vi "AddControlConpane__slk_mt.vi"(8 "error in (no error)":errorcluster, 11 "This VI":refnum<vi>) -> (0 "error IO":errorcluster)   [LabVIEW 2015, in "Lazyboots Menu Tool.lvlib"]
uses:
  <vilib>/SLK/Lazyboots Menu Tool/Library/Lazyboots Menu Tool.lvlib
  <vilib>/Utility/miscctls.llb/LVRectTypeDef.ctl
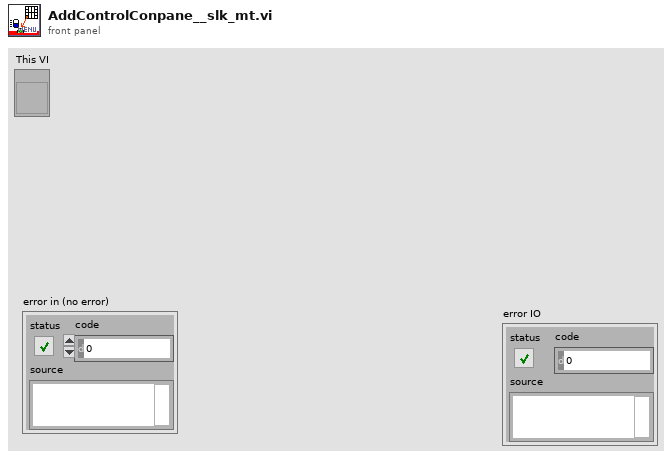
[diagram p1: front panel]
types:
  T1 = typedef "LVRectTypeDef.ctl" = cluster{"Left":i16, "Top":i16, "Right":i16, "Bottom":i16}
  T2 = typedef "LVPositionTypeDef.ctl" = cluster{"Left":i32, "Top":i32}
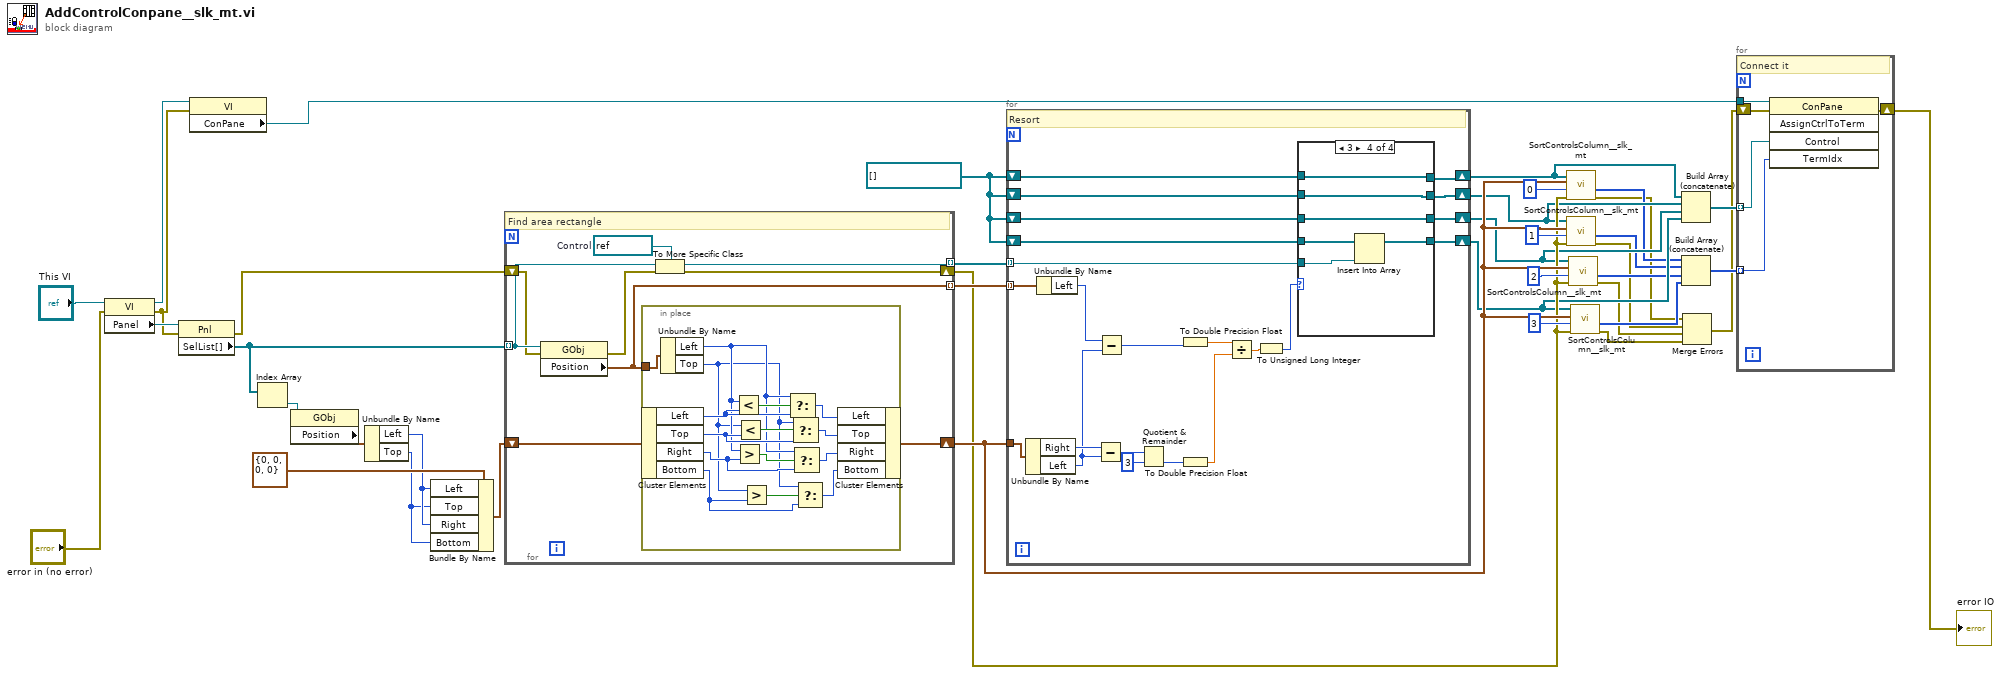
[diagram p0: block diagram]
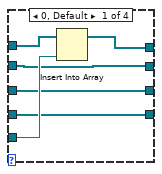
[diagram p2: hidden frame]
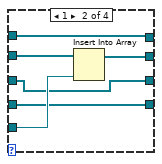
[diagram p3: hidden frame]
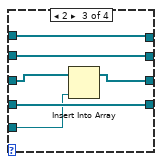
[diagram p4: hidden frame]
diagram:
  w30 = refnum<vi>[] []
  n1 = property class="VI"(reference="This VI", error in="error in (no error)") -> (reference out=w20:refnum<vi>, error out=w19:errorcluster, "Panel"=w21:refnum<vi>)
  n2 = property class="Pnl"(reference=w21, error in=w19) -> (error out=w24:errorcluster, "SelList[]"=w37:refnum<vi>[])  [unwired: 1 out]
  n3 = property class="VI"(reference=w20, error in=w19) -> ("ConPane"=w8:refnum<vi>)  [unwired: 2 out]
  n4 = Index Array(array=w37) -> (element=w36:refnum<vi>)  [unwired: 1 in]
  n5 = property class="GObj"(reference=w36) -> ("Position"=w33:T2)  [unwired: 1 in, 2 out]
  n6 = Unbundle By Name(w33) -> ("Left"=w32:i32, "Top"=w31:i32)
  n7 = Bundle By Name(cluster=T1 {"Left"=0, "Top"=0, "Right"=0, "Bottom"=0} ("Master Bounds Rect"), "Left"=w32, "Top"=w31, "Right"=w32, "Bottom"=w31) -> (w34:T1)
  n8 = for {
    tunnel: w37 -> [w45] mode=indexing
    shift-right: [w47] -> w25
    shift-left: w34 -> [w48]
    tunnel: [w46] -> w38 mode=indexing
    tunnel: [w40] -> w39 mode=indexing
    shift-right: [w41] -> w23
    shift-left: w24 -> [w42]
    w43 = refnum<vi> refnum  # Control
    # "Find area rectangle"
    n9 = property class="GObj"(reference=w45, error in=w42) -> (error out=w44:errorcluster, "Position"=w46:T2)  [unwired: 1 out]
    n10 = in-place {
      in-place-border: w46 -> [w63]
      n11 = in-place-cluster #1(w48) -> ("Left"=w62:i16, "Top"=w58:i16, "Right"=w56:i16, "Bottom"=w50:i16)
      n12 = Unbundle By Name(w63) -> ("Left"=w57:i32, "Top"=w51:i32)
      n13 = Less?(x=w57, y=w62) -> (x < y?=w60:bool)
      n14 = Greater?(x=w57, y=w56) -> (0:w53:bool)
      n15 = Less?(x=w51, y=w58) -> (x < y?=w59:bool)
      n16 = Greater?(x=w51, y=w50) -> (0:w52:bool)
      n17 = Select(t=w57, s=w60, f=w62) -> (s? t:f=w61:i32)
      n18 = Select(t=w51, s=w59, f=w58) -> (s? t:f=w54:i32)
      n19 = Select(t=w57, s=w53, f=w56) -> (s? t:f=w55:i32)
      n20 = Select(t=w51, s=w52, f=w50) -> (s? t:f=w49:i32)
      n21 = in-place-cluster #1("Left"=w61, "Top"=w54, "Right"=w55, "Bottom"=w49) -> (w47:T1)
    }
    n22 = To More Specific Class(target class=w43, reference=w45, error in=w44) -> (specific class reference=w40:refnum<vi>, error out=w41:errorcluster)
  }
  n23 = for {
    tunnel: w39 -> [w74] mode=indexing
    tunnel: w38 -> [w81] mode=indexing
    tunnel: w25 -> [w85]
    shift-right: [w73] -> w18
    shift-left: w30 -> [w78]
    shift-right: [w72] -> w17
    shift-left: w30 -> [w77]
    shift-right: [w71] -> w16
    shift-left: w30 -> [w76]
    shift-right: [w70] -> w15
    shift-left: w30 -> [w75]
    # "Resort"
    n24 = Unbundle By Name(w85) -> ("Right"=w84:i16, "Left"=w79:i16)
    n25 = Unbundle By Name(w81) -> ("Left"=w80:i32)
    n26 = Subtract(x=w84, y=w79) -> (x-y=w83:i16)
    n27 = Subtract(x=w80, y=w79) -> (x-y=w69:i32)
    n28 = Quotient & Remainder(x=w83, y=i16 3) -> (floor(x/y)=w67:i16)  [unwired: 1 out]
    n29 = To Double Precision Float(number=w69) -> (double precision float=w68:dbl)
    n30 = To Double Precision Float(number=w67) -> (double precision float=w66:dbl)
    n31 = Divide(x=w68, y=w66) -> (x/y=w65:dbl)
    n32 = To Unsigned Long Integer(number=w65) -> (unsigned 32bit integer=w64:u32)
    n33 = case shown="3" w64 {
      tunnel: w78 -> [w91 w94 w103 w109]
      tunnel: w77 -> [w88 w97 w101 w105]
      tunnel: w76 -> [w87 w93 w100 w104]
      tunnel: w75 -> [w86 w92 w102 w108]
      tunnel: w74 -> [w90 w96 w98 w106]
      tunnel: [w89 w94 w103 w109] -> w73
      tunnel: [w88 w95 w101 w105] -> w72
      tunnel: [w87 w93 w99 w104] -> w71
      tunnel: [w86 w92 w102 w107] -> w70
      frame 0, Default {
        n34 = Insert Into Array(array=w91, new element=w90) -> (w89:refnum<vi>[])  [unwired: 1 in]
      }
      frame 1 {
        n35 = Insert Into Array(array=w97, new element=w96) -> (w95:refnum<vi>[])  [unwired: 1 in]
      }
      frame 2 {
        n36 = Insert Into Array(array=w100, new element=w98) -> (w99:refnum<vi>[])  [unwired: 1 in]
      }
      frame 3 {
        n37 = Insert Into Array(array=w108, new element=w106) -> (w107:refnum<vi>[])  [unwired: 1 in]
      }
    }
  }
  n38 = call <vilib>:"SortControlsColumn__slk_mt.vi"("error in (no error)"=w23, "Index"=0, "Area Scale"=w25, "Controls"=w18) -> ("error out"=w7:errorcluster, "Index"=w14:u32[])  [unwired: 6 in]
  n39 = call <vilib>:"SortControlsColumn__slk_mt.vi"("error in (no error)"=w23, "Index"=1, "Area Scale"=w25, "Controls"=w17) -> ("error out"=w6:errorcluster, "Index"=w13:u32[])  [unwired: 6 in]
  n40 = call <vilib>:"SortControlsColumn__slk_mt.vi"("error in (no error)"=w23, "Index"=2, "Area Scale"=w25, "Controls"=w16) -> ("error out"=w5:errorcluster, "Index"=w12:u32[])  [unwired: 6 in]
  n41 = call <vilib>:"SortControlsColumn__slk_mt.vi"("error in (no error)"=w23, "Index"=3, "Area Scale"=w25, "Controls"=w15) -> ("error out"=w4:errorcluster, "Index"=w11:u32[])  [unwired: 6 in]
  n42 = Build Array (concatenate)(w18, w17, w16, w15) -> (w10:refnum<vi>[])
  n43 = Build Array (concatenate)(w14, w13, w12, w11) -> (w9:u32[])
  n44 = Merge Errors(w7, w6, w5, w4) -> (w3:errorcluster)
  n45 = for {
    tunnel: w8 -> [w114]
    tunnel: w10 -> [w113] mode=indexing
    tunnel: w9 -> [w112] mode=indexing
    shift-right: [w110] -> w2
    shift-left: w3 -> [w111]
    # "Connect it"
    n46 = invoke class="ConPane" method="AssignCtrlToTerm"(reference=w114, error in=w111, "Control"=w113, "TermIdx"=w112) -> (error out=w110:errorcluster)  [unwired: 1 in, 4 out]
  }
  "error IO" <- w2
